vi "Bed_control_PFITrigger.vi"(8 "Motor speed":string(combo)="Full step", 9 "pulse duration (T/2)":dbl=0.0005 format="%#_13p", 10 "Sequence to run on start up":string[](array[string]), 11 "Signed pulses to move":dbl=50.0) -> ()   [LabVIEW 2021]
uses:
  <vilib>/DAQmx/write.llb/DAQmx Write (Digital 1D Wfm NChan NSamp).vi
  <vilib>/Waveform/DWDTOps.llb/DWDT Digital Size.vi
  Human_Labview/global_variables.vi
  <vilib>/DAQmx/create/channels.llb/DAQmx Create Channel (DO-Digital Output).vi
  <vilib>/DAQmx/configure/timing.llb/DAQmx Timing (Sample Clock).vi
  <vilib>/Waveform/DWDTOps.llb/DWDT Uncompress Digital.vi
  <vilib>/DAQmx/miscellaneous.llb/DAQmx Fill In Error Info.vi
  <vilib>/DAQmx/create/channels.llb/DAQmx Create Channel (CO-Pulse Generation-Frequency).vi
  <vilib>/DAQmx/configure/timing.llb/DAQmx Timing (Implicit).vi
  <resource>/objmgr/daqmx.rc
panel:
  out "x-y":dbl=626.4
  out "-x":dbl=-24.1
  out "Slide":dbl(slide) min=-35.9 max=609.1 scale=-12.9..637.6
  out "Laser:End dist":dbl=626.4
  out "Home:End dist":dbl=650.5
  out "Home:Laser dist":dbl=24.1
  in  "Save Home-Laser Dist":bool
  in  "Sweep":bool
  out "Main loop has stopped":bool
  out "Last system state called":string="Move"
  in  "Read position":bool
  out "Boolean":bool=TRUE
  in  "Number of runs (>1)":i32=3
  out "Bed position":dbl
  out "Application Directory":path=path "C:/Users/MPI/Documents/GitHub/LabviewGUI"
  out "travel distance (mm)":dbl=5.0
  in  "pulse steps":dbl=50.0 min=0.0 step=1.0 format="%#_6p"
  in  "Move bed 2":bool
  out "Homing in progress":bool
  out "duration of movement":dbl=0.05
  in  "Maximum absolute position":i32=60000 format="%.0p"
  out "Absolute position (pulses)":i32=13150
  in  "Abort movement":bool
  in  "Go home!":bool
  in  "Move bed":bool
  in  "Halt":bool
  # "For programatical use only!\nEnsure that the sequence control is empty before setting default values!"
  # "Step 1: Initiate Homing\nStep 2: Physically press ZERO button\nStep 3: Read position\nStep 4: Go to laser position\nStep 5: Read position\nStep 6: Save current position = Laser\nStep 7: Physically press ZERO button"
  # "Homing"
  # "Enables PDU automatically"
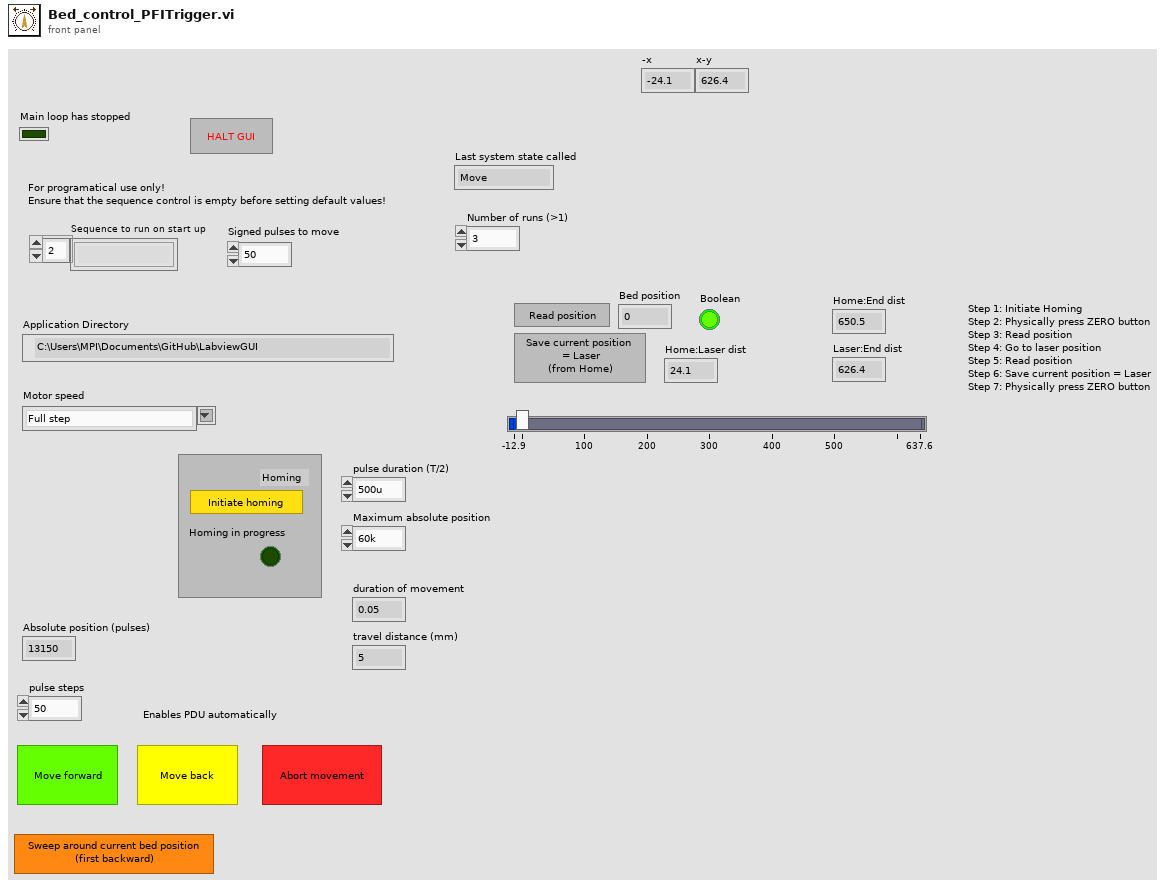
[diagram p1: front panel]
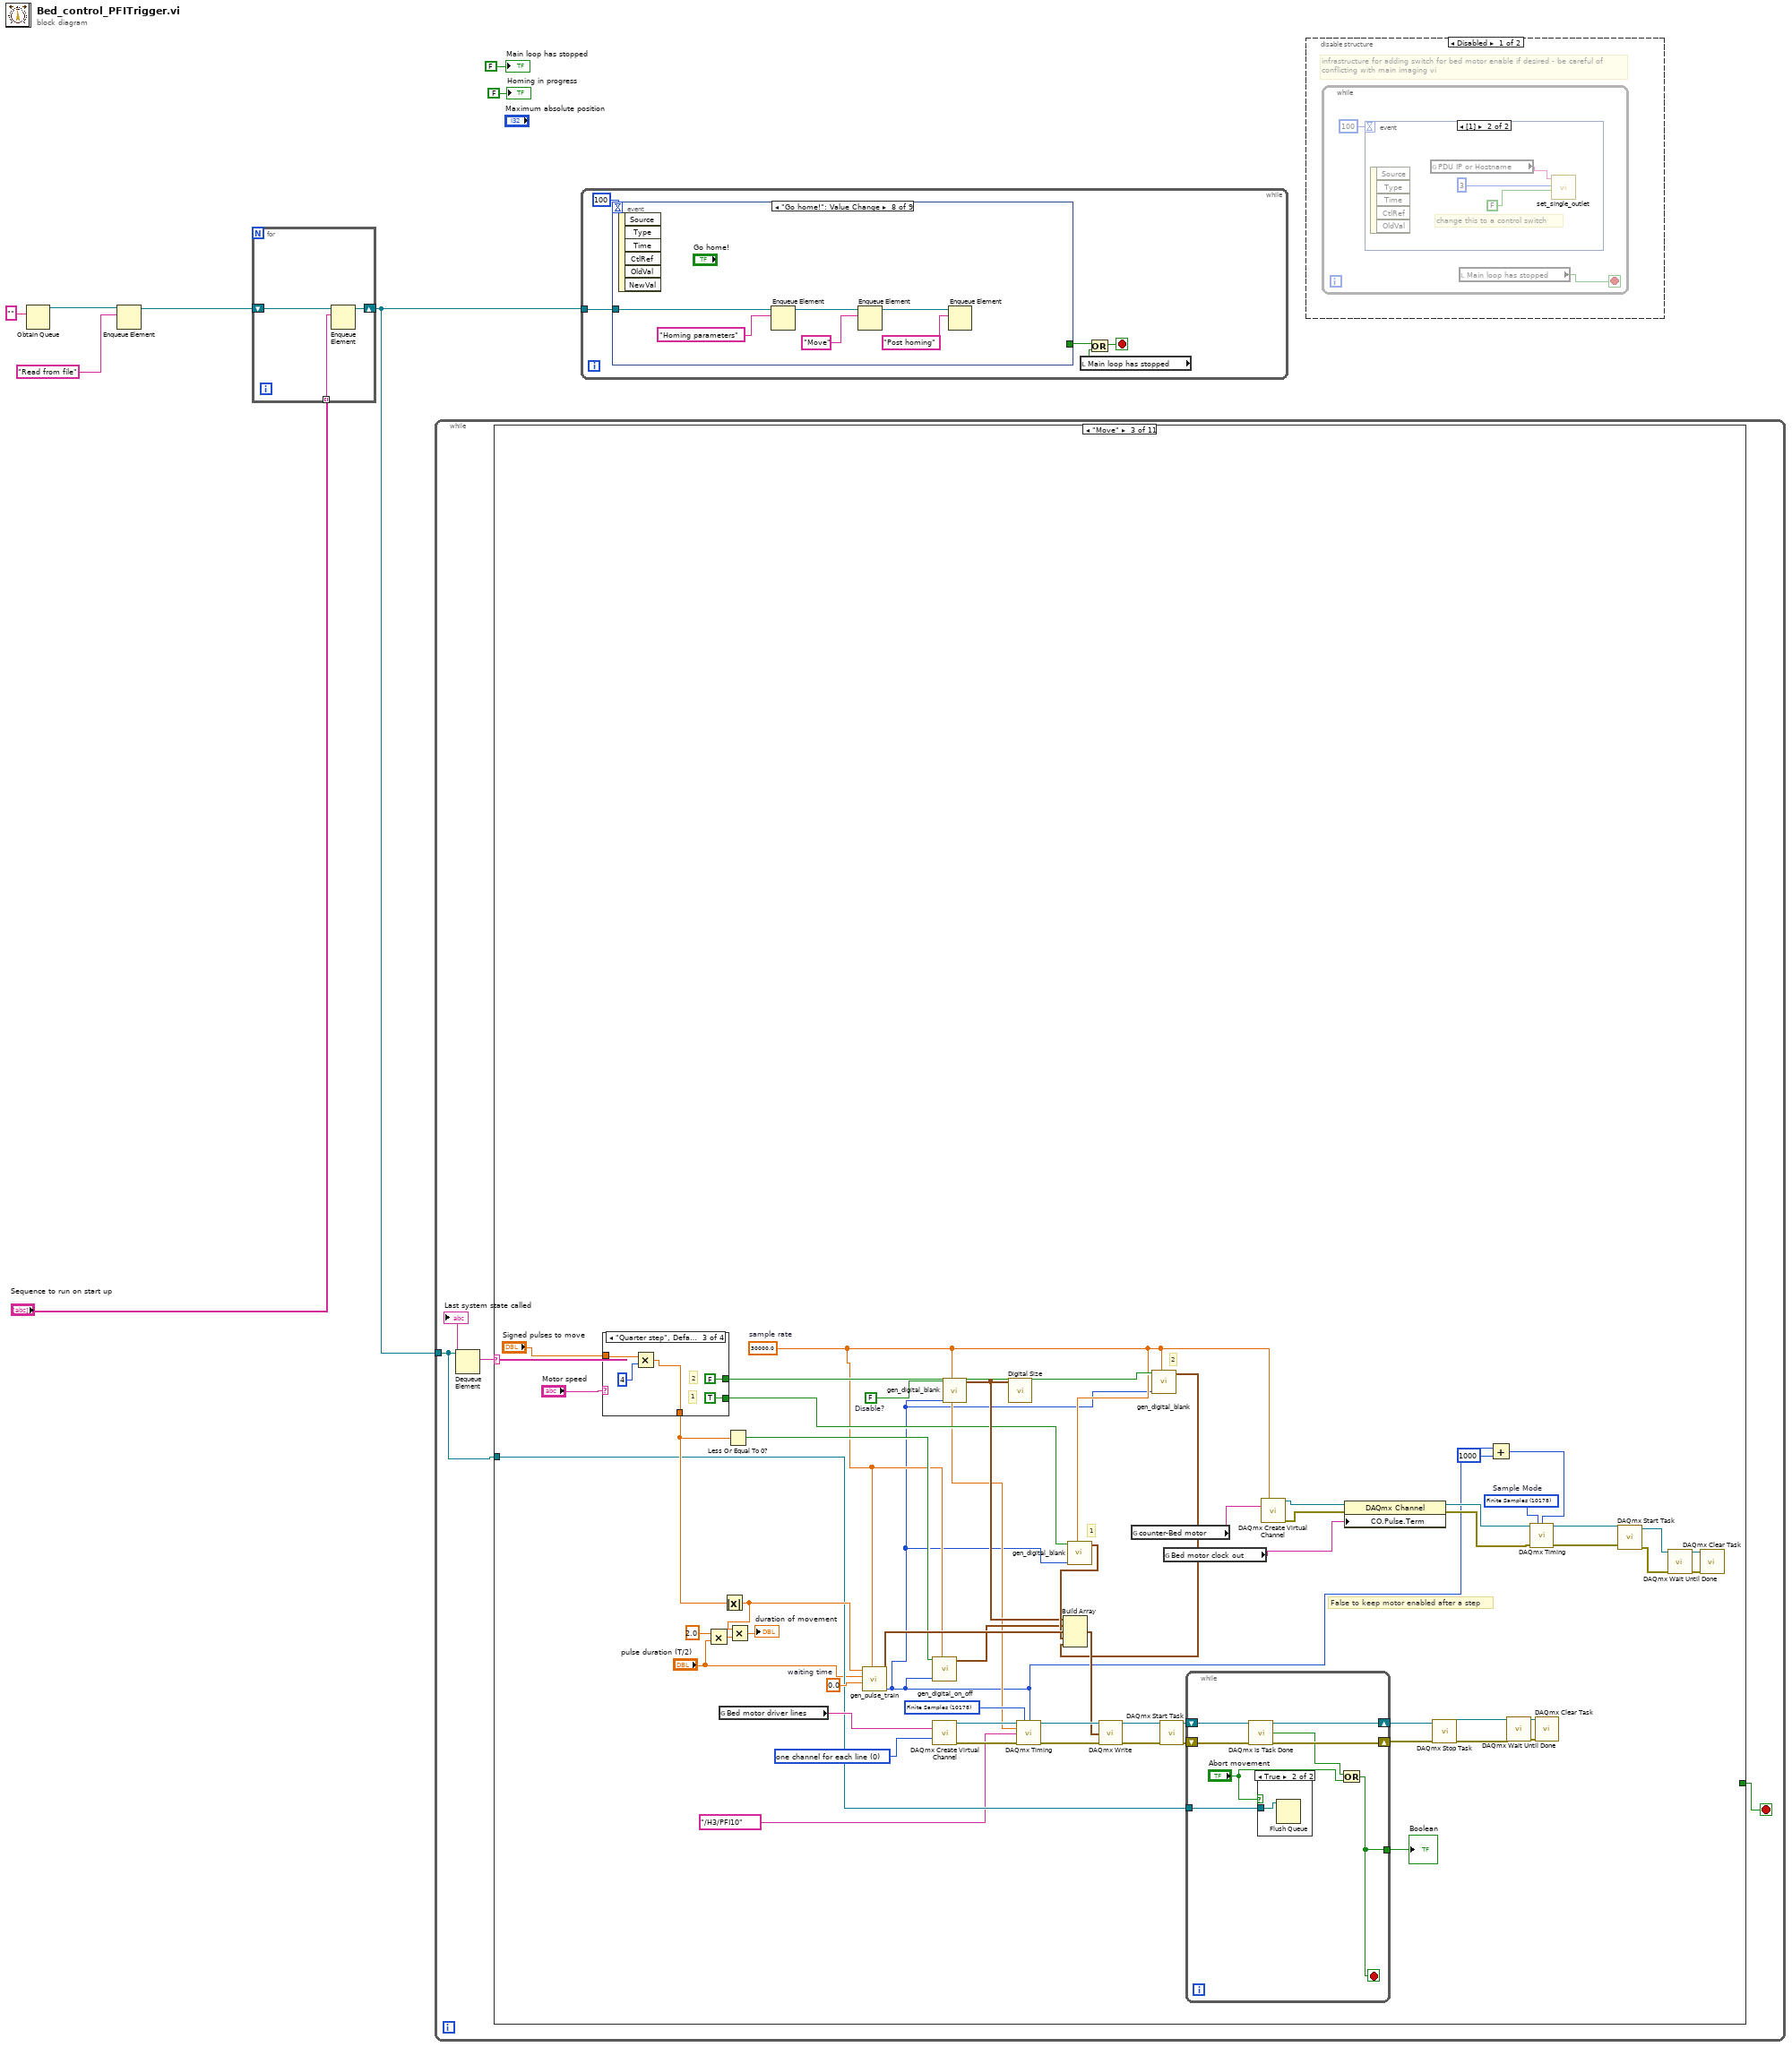
[diagram p0: block diagram]
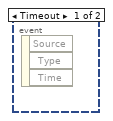
[diagram p2: hidden frame]
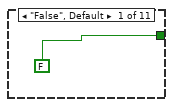
[diagram p4: hidden frame]
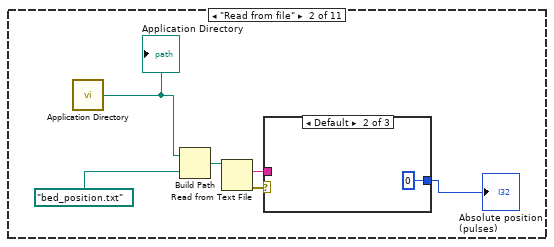
[diagram p5: hidden frame]
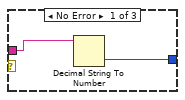
[diagram p6: hidden frame]
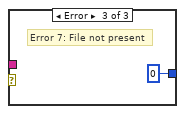
[diagram p7: hidden frame]
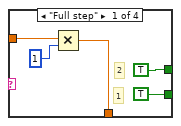
[diagram p8: hidden frame]
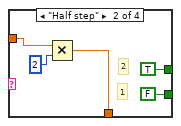
[diagram p9: hidden frame]
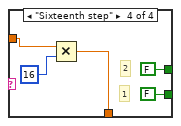
[diagram p10: hidden frame]
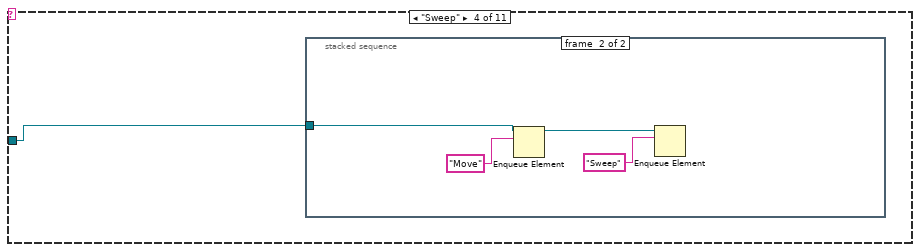
[diagram p12: hidden frame]
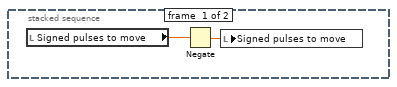
[diagram p13: hidden frame]
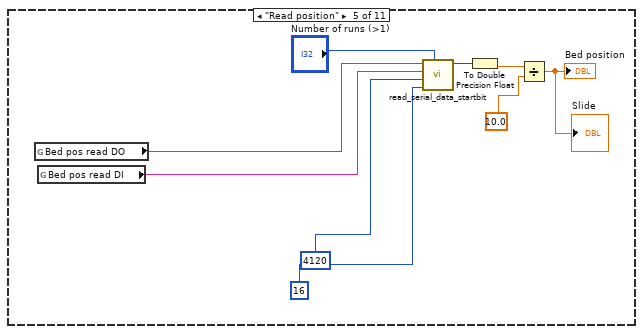
[diagram p14: hidden frame]
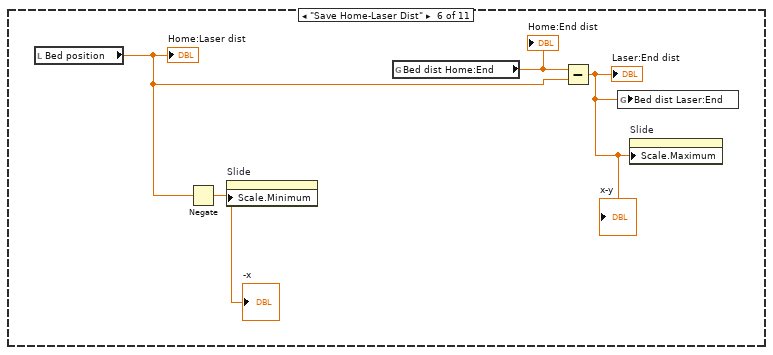
[diagram p15: hidden frame]
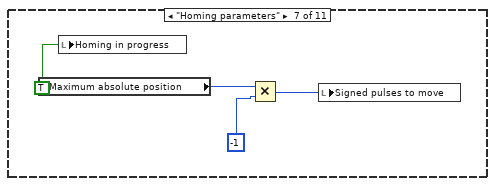
[diagram p16: hidden frame]
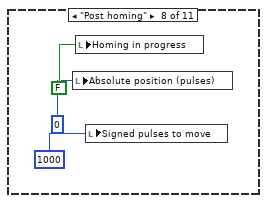
[diagram p17: hidden frame]
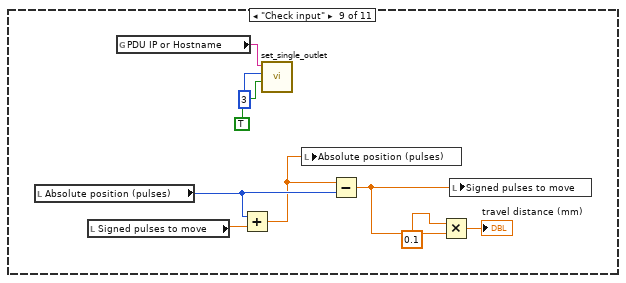
[diagram p18: hidden frame]
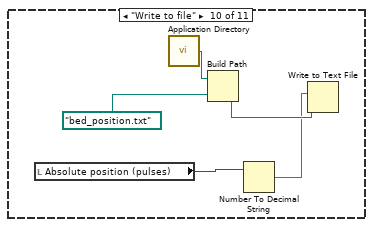
[diagram p19: hidden frame]
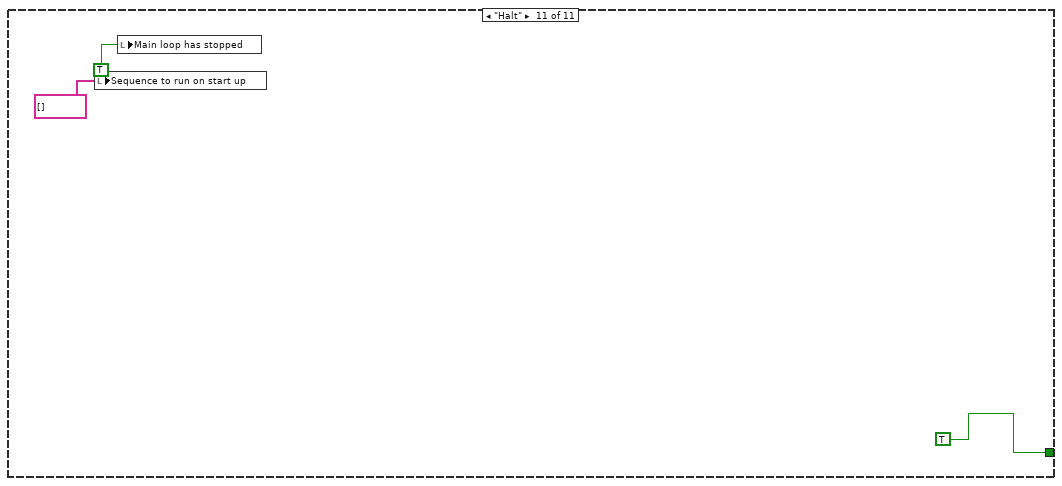
[diagram p20: hidden frame]
diagram:
  n1 = Obtain Queue(element data type="") -> (queue out=w7:refnum<queue>)  [unwired: 4 in, 2 out]
  n2 = Enqueue Element(queue=w7, element="Read from file") -> (queue out=w4:refnum<queue>)  [unwired: 2 in, 2 out]
  n3 = for {
    shift-right: [w10] -> w3
    shift-left: w4 -> [w11]
    tunnel: "Sequence to run on start up" -> [w9] mode=indexing
    n4 = Enqueue Element(queue=w11, element=w9) -> (queue out=w10:refnum<queue>)  [unwired: 2 in, 2 out]
  }
  n5 = while {
    tunnel: w3 -> [w12]
    stop <- w13 stop-if-true
    n6 = Dequeue Element(queue=w12) -> (element=w14:string)  [unwired: 2 in, 3 out]
    "Last system state called" <- w14
    n7 = case shown="\"Move\"" w14 {
      tunnel: [FALSE _ _ _ _ _ _ _ _ _ TRUE] -> w13
      tunnel: w12 -> [_ _ w48 w111 _ _ _ _ _ _ _]
      frame "False", Default {
      }
      frame "Read from file" {
        n8 = call <vilib>:"Application Directory.vi"() -> ("Application Directory"=w18:path)
        "Application Directory" <- w18
        n9 = Build Path(base path=w18, name or relative path=path "bed_position.txt" ("file (use dialog)")) -> (appended path=w19:path)
        n10 = Read from Text File(file (use dialog)=w19) -> (text=w21:string, error out=w20:errorcluster)  [unwired: 3 in, 2 out]
        n11 = case shown="Default" w20 {
          tunnel: w21 -> [w23 _ _]
          tunnel: [w22 0 0] -> w16
          frame No Error {
            n12 = Decimal String To Number(string=w23) -> (number=w22:i32)  [unwired: 2 in, 1 out]
          }
          frame Default {
          }
          frame Error {
            # "Error 7: File not present"
          }
        }
        "Absolute position (pulses)" <- w16
      }
      frame "Move" {
        w39 = 10178 items=["Finite Samples"=10178, "Continuous Samples"=10123, "Hardware Timed Single Point"=12522]  # Sample Mode
        w71 = 0.0  # waiting time
        w37 = 30000.0  # sample rate
        w74 = FALSE  # Disable?
        w73 = 10178 items=["Finite Samples"=10178, "Continuous Samples"=10123, "Hardware Timed Single Point"=12522] ("sample mode")
        w72 = 0 items=["one channel for each line", "one channel for all lines"] ("line grouping")
        # "1"
        # "2"
        # "False to keep motor enabled after a step"
        n13 = case shown="\"Quarter step\", Default" "Motor speed" {
          tunnel: "Signed pulses to move" -> [w85 w90 w95 w100]
          tunnel: [TRUE ("motor speed control 1") TRUE ("motor speed control 1") FALSE ("motor speed control 1") FALSE ("motor speed control 1")] -> w53
          tunnel: [TRUE ("motor speed control 1") FALSE ("motor speed control 1") TRUE ("motor speed control 1") FALSE ("motor speed control 1")] -> w52
          tunnel: [w82 w87 w92 w97] -> w51
          frame "Full step" {
            # "1"
            # "2"
            n14 = Multiply(x=w85, y=1) -> (x*y=w82:dbl)
          }
          frame "Half step" {
            # "1"
            # "2"
            n15 = Multiply(x=w90, y=2) -> (x*y=w87:dbl)
          }
          frame "Quarter step", Default {
            # "1"
            # "2"
            n16 = Multiply(x=w95, y=4) -> (x*y=w92:dbl)
          }
          frame "Sixteenth step" {
            # "1"
            # "2"
            n17 = Multiply(x=w100, y=16) -> (x*y=w97:dbl)
          }
        }
        n18 = Multiply(x=2.0, y="pulse duration (T/2)") -> (x*y=w67:dbl)
        n19 = global read "global_variables.vi" "Bed motor driver lines"() -> (w50:tag)
        n20 = Absolute Value(x=w51) -> (abs(x)=w68:dbl)
        n21 = Less Or Equal To 0?(x=w51) -> (x <= 0?=w70:bool)
        n22 = Multiply(x=w68, y=w67) -> (x*y=→"duration of movement":dbl)
        n23 = call "gen_pulse_train.vi"("sampling rate"=w37, "waiting time"=w71, "pulse width"="pulse duration (T/2)", "Number of pulses"=w68) -> ("waveform length"=w28:i32, "digital waveform out"=w79:digitalwaveform)  [unwired: 6 in]
        n24 = call "gen_digital_on_off.vi"("sampling rate"=w37, "waveform length"=w28, "On / Off"=w70) -> ("digital waveform"=w55:digitalwaveform)  [unwired: 8 in]
        n25 = call-poly <vilib>:"DAQmx Create Virtual Channel.vi"("lines"=w50, "line grouping"=w72) -> ("task out"=w75:refnum<k21>, "error out"=w78:errorcluster)  [unwired: 12 in]
        n26 = call "gen_digital_blank.vi"("sampling rate"=w37, "waveform length"=w28, "On / Off"=w74) -> ("digital waveform"=w56:digitalwaveform)  [unwired: 8 in]
        n27 = call-poly <vilib>:"Digital Size.vi"("digital waveform in"=w56) -> ()  [unwired: 7 in, 4 out]
        n28 = call-poly <vilib>:"DAQmx Timing.vi"("task/channels in"=w75, "sample mode"=w73, "samples per channel"=w28, "rate"=w37, "source"=tag "/H3/PFI10", "error in"=w78) -> ("task out"=w76:refnum<k21>, "error out"=w77:errorcluster)  [unwired: 8 in]
        n29 = call "gen_digital_blank.vi"("sampling rate"=w37, "waveform length"=w28, "On / Off"=w52) -> ("digital waveform"=w57:digitalwaveform)  [unwired: 8 in]
        n30 = global read "global_variables.vi" "counter-Bed motor"() -> (w46:tag)
        n31 = call "gen_digital_blank.vi"("sampling rate"=w37, "waveform length"=w28, "On / Off"=w53) -> ("digital waveform"=w58:digitalwaveform)  [unwired: 8 in]
        n32 = Build Array(w56, w55, w79, w57, w58) -> (w59:digitalwaveform[])
        n33 = call-poly <vilib>:"DAQmx Write.vi"("task/channels in"=w76, "data"=w59, "error in"=w77) -> ("task out"=w80:refnum<k21>, "error out"=w81:errorcluster)  [unwired: 10 in, 1 out]
        n34 = call <vilib>:"DAQmx Start Task.vi"("task/channels in"=w80, "error in"=w81) -> ("task out"=w65:refnum<k21>, "error out"=w64:errorcluster)  [unwired: 12 in]
        n35 = global read "global_variables.vi" "Bed motor clock out"() -> (w47:tag)
        n36 = while {
          shift-right: [w106] -> w62
          shift-left: w64 -> [w108]
          shift-right: [w107] -> w63
          shift-left: w65 -> [w109]
          tunnel: w48 -> [w105]
          tunnel: [w102] -> w29
          stop <- w102 stop-if-true
          n37 = call <vilib>:"DAQmx Is Task Done.vi"("task/channels in"=w109, "error in"=w108) -> ("task out"=w107:refnum<k21>, "task done?"=w104:bool, "error out"=w106:errorcluster)  [unwired: 11 in]
          n38 = case shown="True" "Abort movement" {
            tunnel: w105 -> [_ w110]
            frame False {
            }
            frame True {
              n39 = Flush Queue(queue=w110) -> ()  [unwired: 1 in, 3 out]
            }
          }
          n40 = Or(x=w104, y="Abort movement") -> (x .or. y?=w102:bool)
        }
        "Boolean" <- w29
        n41 = call-poly <vilib>:"DAQmx Create Virtual Channel.vi"("frequency"=w37, "counter"=w46) -> ("task out"=w45:refnum<k21>, "error out"=w44:errorcluster)  [unwired: 12 in]
        n42 = property class="DAQmx Channel"(reference=w45, error in=w44, "CO.Pulse.Term"=w47) -> (reference out=w43:refnum<k21>, error out=w42:errorcluster)
        n43 = call <vilib>:"DAQmx Stop Task.vi"("task/channels in"=w63, "error in"=w62) -> ("task out"=w32:refnum<k21>, "error out"=w31:errorcluster)  [unwired: 12 in]
        n44 = Add(x=w28, y=1000) -> (x+y=w27:i32)
        n45 = call <vilib>:"DAQmx Wait Until Done.vi"("task/channels in"=w32, "error in"=w31) -> ("task out"=w61:refnum<k21>, "error out"=w60:errorcluster)  [unwired: 12 in]
        n46 = call-poly <vilib>:"DAQmx Timing.vi"("task/channels in"=w43, "sample mode"=w39, "samples per channel"=w27, "error in"=w42) -> ("task out"=w40:refnum<k21>, "error out"=w41:errorcluster)  [unwired: 10 in]
        n47 = call <vilib>:"DAQmx Clear Task.vi"("task in"=w61, "error in"=w60) -> ()  [unwired: 13 in, 1 out]
        n48 = call <vilib>:"DAQmx Start Task.vi"("task/channels in"=w40, "error in"=w41) -> ("task out"=w33:refnum<k21>, "error out"=w30:errorcluster)  [unwired: 12 in]
        n49 = call <vilib>:"DAQmx Wait Until Done.vi"("task/channels in"=w33, "error in"=w30) -> ("task out"=w34:refnum<k21>, "error out"=w35:errorcluster)  [unwired: 12 in]
        n50 = call <vilib>:"DAQmx Clear Task.vi"("task in"=w34, "error in"=w35) -> ()  [unwired: 13 in, 1 out]
      }
      frame "Sweep" {
        n51 = stacked-sequence {
          tunnel: w111 -> [_ w116]
          frame #0 {
            n52 = local read "Signed pulses to move"() -> (w113:dbl)
            n53 = Negate(x=w113) -> (-x=w112:dbl)
            n54 = local write "Signed pulses to move"(w112) -> ()
          }
          frame #1 {
            n55 = Enqueue Element(queue=w116, element="Move") -> (queue out=w114:refnum<queue>)  [unwired: 2 in, 2 out]
            n56 = Enqueue Element(queue=w114, element="Sweep") -> ()  [unwired: 2 in, 3 out]
          }
        }
      }
      frame "Read position" {
        n57 = global read "global_variables.vi" "Bed pos read DO"() -> (w122:tag)
        n58 = global read "global_variables.vi" "Bed pos read DI"() -> (w121:tag)
        n59 = call "read_serial_data_startbit.vi"("Number of runs"="Number of runs (>1)", "No. expected bits"=u16 16, "baud rate"=u32 4120, "Digital input line"=w121, "Digital output line"=w122) -> ("mode"=w126:i16)  [unwired: 4 in, 1 out]
        n60 = To Double Precision Float(number=w126) -> (double precision float=w124:dbl)
        n61 = Divide(x=w124, y=10.0) -> (x/y=→"Bed position" →"Slide":dbl)
      }
      frame "Save Home-Laser Dist" {
        n62 = local read "Bed position"() -> (w129:dbl)
        "Home:Laser dist" <- w129
        n63 = Negate(x=w129) -> (-x=w128:dbl)
        "-x" <- w128
        n64 = property on="Slide" class="Slide (strict)"("Scale.Minimum"=w128) -> ()  [unwired: 2 in, 2 out]
        n65 = global read "global_variables.vi" "Bed dist Home:End"() -> (w130:dbl)
        "Home:End dist" <- w130
        n66 = Subtract(x=w130, y=w129) -> (x-y=w127:dbl)
        "Laser:End dist" <- w127
        "x-y" <- w127
        n67 = global write "global_variables.vi" "Bed dist Laser:End"(w127) -> ()
        n68 = property on="Slide" class="Slide (strict)"("Scale.Maximum"=w127) -> ()  [unwired: 2 in, 2 out]
      }
      frame "Homing parameters" {
        n69 = local read "Maximum absolute position"() -> (w133:i32)
        n70 = local write "Homing in progress"(TRUE ("Homing in progress")) -> ()
        n71 = Multiply(x=w133, y=-1) -> (x*y=w131:i32)
        n72 = local write "Signed pulses to move"(w131) -> ()
      }
      frame "Post homing" {
        n73 = local write "Absolute position (pulses)"(0 ("Absolute position (pulses)")) -> ()
        n74 = local write "Homing in progress"(FALSE ("Homing in progress")) -> ()
        n75 = local write "Signed pulses to move"(1000 ("pulses to move")) -> ()
      }
      frame "Check input" {
        n76 = local read "Absolute position (pulses)"() -> (w146:i32)
        n77 = local read "Signed pulses to move"() -> (w139:dbl)
        n78 = global read "global_variables.vi" "PDU IP or Hostname"() -> (w142:string)
        n79 = Add(x=w146, y=w139) -> (x+y=w138:dbl)
        n80 = call "set_single_outlet.vi"("Switch state"=TRUE, "Outlet #"=3, "IP / Hostname"=w142) -> ()  [unwired: 9 in]
        n81 = local write "Absolute position (pulses)"(w138) -> ()
        n82 = Subtract(x=w138, y=w146) -> (x-y=w143:dbl)
        n83 = Multiply(x=0.1, y=w143) -> (x*y=→"travel distance (mm)":dbl)
        n84 = local write "Signed pulses to move"(w143) -> ()
      }
      frame "Write to file" {
        n85 = local read "Absolute position (pulses)"() -> (w147:i32)
        n86 = call <vilib>:"Application Directory.vi"() -> ("Application Directory"=w151:path)
        n87 = Build Path(base path=w151, name or relative path=path "bed_position.txt" ("file (use dialog)")) -> (appended path=w150:path)
        n88 = Number To Decimal String(number=w147) -> (decimal integer string=w149:string)  [unwired: 1 in]
        n89 = Write to Text File(file (use dialog)=w150, text=w149) -> ()  [unwired: 2 in, 3 out]
      }
      frame "Halt" {
        n90 = local write "Sequence to run on start up"(string[] [] ("Sequence to run on start up")) -> ()
        n91 = local write "Main loop has stopped"(TRUE ("Main loop has stopped")) -> ()
      }
    }
  }
  n92 = while {
    tunnel: w3 -> [w159]
    stop <- w156 stop-if-true
    n93 = event shown="[7] \"Go home!\": Value Change" {
      selector: _ -> [_ _ _ _ _ _ _ _ _]
      dyn-events: _ -> [_ _ _ _ _ _ _ _ _]
      timeout: 100 -> [_ _ _ _ _ _ _ _ _]
      tunnel: w159 -> [_ w163 w164 w170 _ w174 w183 w189 w192]
      tunnel: [FALSE TRUE _ _ _ _ _ _ _] -> w157
      event Timeout {
        n94 = event-data() -> ()  [unwired: 1 in, 3 out]
      }
      event "Halt": Value Change {
        n95 = event-data() -> ()  [unwired: 1 in, 6 out]
        n96 = Enqueue Element(queue=w163, element="Halt") -> ()  [unwired: 2 in, 3 out]
      }
      event "Move bed": Value Change {
        n97 = event-data() -> ()  [unwired: 1 in, 6 out]
        n98 = stacked-sequence {
          tunnel: w164 -> [_ w166]
          frame #0 {
            n99 = local write "Signed pulses to move"("pulse steps") -> ()
          }
          frame #1 {
            n100 = Enqueue Element(queue=w166, element="Check input") -> (queue out=w167:refnum<queue>)  [unwired: 2 in, 2 out]
            n101 = Enqueue Element(queue=w167, element="Move") -> ()  [unwired: 2 in, 3 out]
          }
        }
      }
      event "Sweep": Value Change {
        n102 = event-data() -> ()  [unwired: 1 in, 6 out]
        n103 = stacked-sequence {
          tunnel: w170 -> [_ w172]
          frame #0 {
            n104 = local read "pulse steps"() -> (w171:dbl)
            n105 = local write "Signed pulses to move"(w171) -> ()
          }
          frame #1 {
            n106 = Enqueue Element(queue=w172, element="Sweep") -> ()  [unwired: 2 in, 3 out]
          }
        }
      }
      event Key Down? {
        n107 = event-data() -> ()  [unwired: 1 in, 10 out]
        n108 = event-data() -> ()  [unwired: 7 in, 1 out]
      }
      event "Move bed 2": Value Change {
        n109 = event-data() -> ()  [unwired: 1 in, 6 out]
        n110 = stacked-sequence {
          tunnel: w174 -> [_ w177]
          frame #0 {
            n111 = local read "pulse steps"() -> (w175:dbl)
            n112 = Negate(x=w175) -> (-x=w176:dbl)
            n113 = local write "Signed pulses to move"(w176) -> ()
          }
          frame #1 {
            n114 = Enqueue Element(queue=w177, element="Check input") -> (queue out=w178:refnum<queue>)  [unwired: 2 in, 2 out]
            n115 = Enqueue Element(queue=w178, element="Move") -> ()  [unwired: 2 in, 3 out]
          }
        }
      }
      event "Save Home-Laser Dist": Value Change {
        n116 = event-data() -> ()  [unwired: 1 in, 6 out]
        n117 = Enqueue Element(queue=w183, element="Read position") -> (queue out=w181:refnum<queue>)  [unwired: 2 in, 2 out]
        n118 = Enqueue Element(queue=w181, element="Save Home-Laser Dist") -> ()  [unwired: 2 in, 3 out]
      }
      event "Go home!": Value Change {
        n119 = event-data() -> ()  [unwired: 1 in, 6 out]
        n120 = Enqueue Element(queue=w189, element="Homing parameters") -> (queue out=w187:refnum<queue>)  [unwired: 2 in, 2 out]
        n121 = Enqueue Element(queue=w187, element="Move") -> (queue out=w185:refnum<queue>)  [unwired: 2 in, 2 out]
        n122 = Enqueue Element(queue=w185, element="Post homing") -> ()  [unwired: 2 in, 3 out]
      }
      event "Read position": Value Change {
        n123 = event-data() -> ()  [unwired: 1 in, 6 out]
        n124 = Enqueue Element(queue=w192, element="Read position") -> ()  [unwired: 2 in, 3 out]
      }
    }
    n125 = local read "Main loop has stopped"() -> (w158:bool)
    n126 = Or(x=w157, y=w158) -> (x .or. y?=w156:bool)
  }
  n127 = disable-structure shown="Disabled" {
    frame Disabled {
      # "infrastructure for adding switch for bed motor enable if desired - be careful of conflicting with main imaging vi"
      n128 = while {
        stop <- w193 stop-if-true
        n129 = event shown="[1]" {
          selector: _ -> [_ _]
          dyn-events: _ -> [_ _]
          timeout: 100 -> [_ _]
          event Timeout {
            n130 = event-data() -> ()  [unwired: 1 in, 3 out]
          }
          event #1 (no event record) {
            # "change this to a control switch"
            n131 = event-data() -> ()  [unwired: 1 in, 5 out]
            n132 = global read "global_variables.vi" "PDU IP or Hostname"() -> (w197:string)
            n133 = call "set_single_outlet.vi"("Switch state"=FALSE, "Outlet #"=3, "IP / Hostname"=w197) -> ()  [unwired: 9 in]
          }
        }
        n134 = local read "Main loop has stopped"() -> (w193:bool)
      }
    }
    frame Enabled {
    }
  }
  "Homing in progress" <- FALSE ("Homing in progress")
  "Main loop has stopped" <- FALSE ("Main loop has stopped")
